vi "spec_GetOpticalExitPort.vi"(8 "error in (no error)":errorcluster, 11 "LightField Automation in":refnum<class "LightField Automation.lvclass">) -> (0 "error out":errorcluster, 2 "Exit Port Location":T1 items=["None"=1, "SideEntrance"=2, "FrontEntrance"=3, "SideExit"=5, "FrontExit"=4], 3 "LightField Automation out":refnum<class "LightField Automation.lvclass">)   [LabVIEW 2020, in "LightField Automation.lvclass"]
uses:
  LightField Automation.lvclass
  TypeDefs/OpticalPortLocation.ctl
  C:/Program Files/Princeton Instruments/LightField/PrincetonInstruments.LightFieldAddInSupportServices.dll
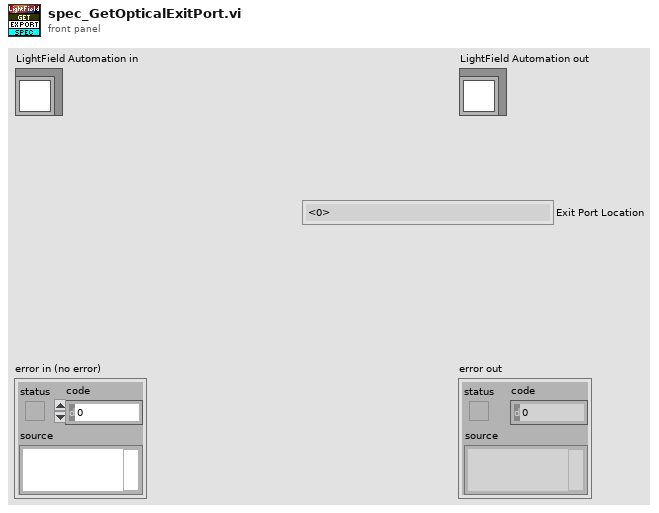
[diagram p1: front panel]
types:
  T1 = typedef "LightField Automation.lvclass/OpticalPortLocation.ctl" = i32
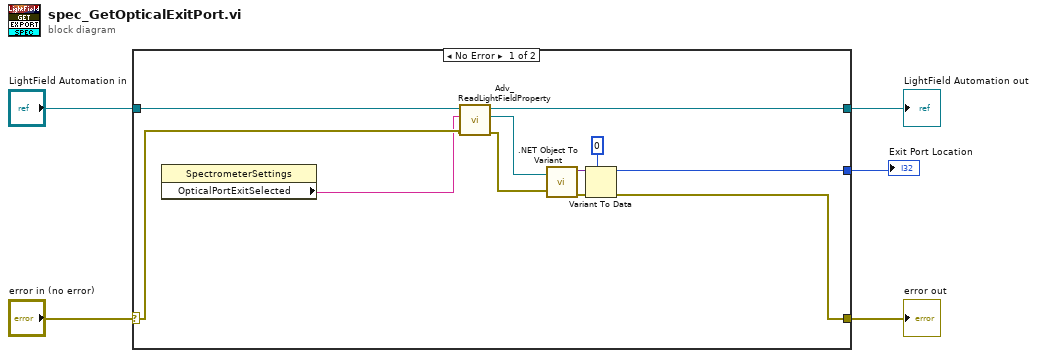
[diagram p0: block diagram]
diagram:
  n1 = case shown="No Error" "error in (no error)" {
    selector: "error in (no error)" -> [w9 w18]
    tunnel: [w7 w18] -> w4
    tunnel: [w11 w17] -> w2
    tunnel: "LightField Automation in" -> [w10 w17]
    tunnel: [w6 _] -> w1
    frame No Error {
      n2 = property class="SpectrometerSettings"() -> ("OpticalPortExitSelected"=w8:string)  [unwired: 2 in, 2 out]
      n3 = call "Adv_ReadLightFieldProperty.vi"("error in (no error)"=w9, "setting"=w8, "LightField Automation in"=w10) -> ("error out"=w15:errorcluster, "value"=w16:refnum<k24>, "LightField Automation out"=w11:refnum<class "LightField Automation.lvclass">)  [unwired: 6 in]
      n4 = call <vilib>:".NET Object To Variant.vi"("error in (no error)"=w15, ".NET object"=w16) -> ("error out"=w12:errorcluster, "variant"=w14:variant)
      n5 = Variant To Data(error in=w12, type=0, Variant=w14) -> (data=w6:i32, error out=w7:errorcluster)
    }
    frame Error {
    }
  }
  "error out" <- w4
  "LightField Automation out" <- w2
  "Exit Port Location" <- w1
